vi "Tektronix AFG 3000 Series Generate Arbitrary Waveform.vi"() -> ()   [LabVIEW 2017, in "Tektronix AFG 3000 Series.lvlib"]
doc: "Demonstrates how to configure then create an arbitrary waveform."
uses:
  Tektronix AFG 3000 Series.lvlib
  Instance           1 61Saved   Tektronix AFG 3000 Series Generate Arbitrary Waveform .vi
  Instance           2 61Saved   Tektronix AFG 3000 Series Generate Arbitrary Waveform .vi
panel:
  in  "Frequency (1000 Hz)":dbl[unit]=1000.0
  in  "DC Offset (0 V)":dbl[unit]
  in  "Gain (1 V)":dbl[unit]=1.0
  in  "Arbitrary Waveform Name (0: USER1)":u16(ring) items=["USER1", "USER2", "USER3", "USER4"]
  in  "Channel (0: Channel 1)":u16(ring) items=["Channel 1", "Channel 2"]
  in  "VISA resource name":refnum<visa-resource-name>
  # "(c) 2006-2009 National Instruments.  ALL RIGHTS RESERVED."
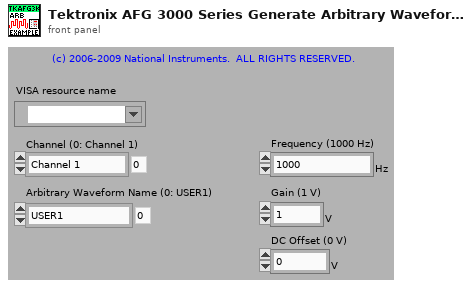
[diagram p1: front panel]
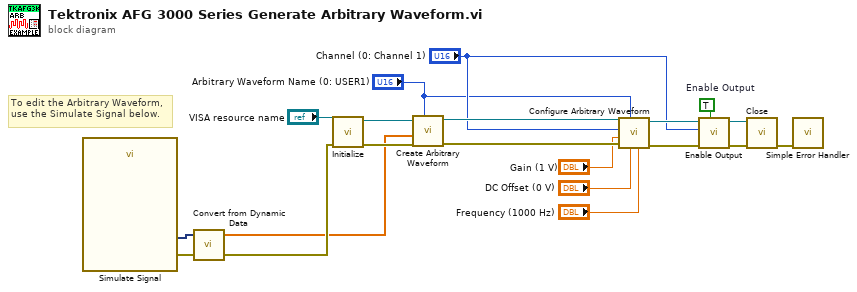
[diagram p0: block diagram]
diagram:
  w8 = TRUE  # Enable Output
  # "To edit the Arbitrary Waveform, use the Simulate Signal below."
  n1 = call "Simulate Signal"() -> ("Sine with Uniform Noise"=w10:dynamicdata, "error out"=w11:errorcluster)  [unwired: 8 in, 6 out]
  n2 = call "Convert from Dynamic Data"("Dynamic Data Type"=w10) -> ("Array"=w6:dbl[])  [unwired: 3 out]
  n3 = call "Initialize.vi"("error in (no error)"=w11, "VISA resource name"="VISA resource name") -> ("error out"=w12:errorcluster, "VISA resource name out"=w7:refnum<visa-resource-name>)  [unwired: 2 in, 6 out]
  n4 = call "Create Arbitrary Waveform.vi"("Arbitrary Waveform Name (0: USER1)"="Arbitrary Waveform Name (0: USER1)", "error in (no error)"=w12, "Arbitrary Waveform Data"=w6, "VISA resource name"=w7) -> ("error out"=w14:errorcluster, "VISA resource name out"=w15:refnum<visa-resource-name>)  [unwired: 1 in, 5 out]
  n5 = call "Configure Arbitrary Waveform.vi"("Frequency (1000 Hz)"="Frequency (1000 Hz)", "DC Offset (0 V)"="DC Offset (0 V)", "Arbitrary Waveform Name (0: USER1)"="Arbitrary Waveform Name (0: USER1)", "error in (no error)"=w14, "Gain (1 V)"="Gain (1 V)", "Channel (0: Channel 1)"="Channel (0: Channel 1)", "VISA resource name"=w15) -> ("error out"=w13:errorcluster, "VISA resource name out"=w16:refnum<visa-resource-name>)  [unwired: 1 in, 2 out]
  n6 = call "Enable Output.vi"("Enable Output (T: Enable)"=w8, "error in (no error)"=w13, "Channel (0: Channel 1)"="Channel (0: Channel 1)", "VISA resource name"=w16) -> ("error out"=w17:errorcluster, "VISA resource name out"=w18:refnum<visa-resource-name>)  [unwired: 6 out]
  n7 = call "Close.vi"("error in (no error)"=w17, "VISA resource name"=w18) -> ("error out"=w19:errorcluster)  [unwired: 9 out]
  n8 = call <vilib>:"Simple Error Handler.vi"("error in (no error)"=w19) -> ()  [unwired: 1 in, 8 out]
